vi "Voice Level Processing.vi"(8 "error in (no error)":errorcluster, 9 "Signal Generation in":variant, 10 "Voice Level Controls in":variant, 11 "MIDI Controls in":variant) -> (0 "error out":errorcluster, 2 "Voice Level Processing out":variant)   [LabVIEW 2014, in "mySynthesizer.lvlib" / "Voice Level Processing.lvlib"]
uses:
  Voice Level Processing.lvlib
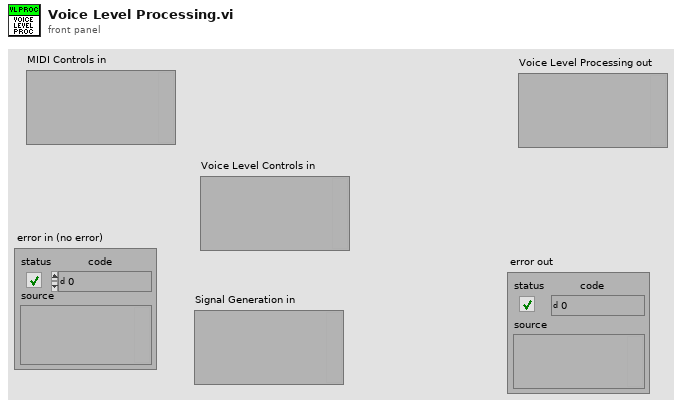
[diagram p1: front panel]
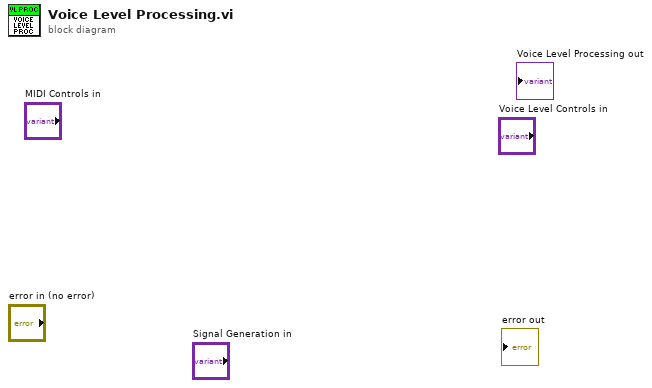
[diagram p0: block diagram]
diagram:
